vi "Change Type.vi"(8 "error in (no error)":errorcluster, 10 "Type":i32(listbox), 11 "Numeric Data Type in":refnum<class "Numeric Data Type.lvclass">) -> (0 "error out":errorcluster, 3 "Numeric Data Type out":refnum<class "Numeric Data Type.lvclass">)   [LabVIEW 2018, in "Numeric Data Type.lvclass"]
uses:
  Numeric Data Type.lvclass
  Numeric Format Enum.ctl
  Numeric Data Type.lvclass/Numeric Data Type.ctl
  Numeric Info.ctl
  Precision Type.ctl
  Padding.ctl
  Time Info.ctl
  Time Format.ctl
  Clock Type.ctl
  Date Order.ctl
  Date Format.ctl
  Year Format.ctl
  Format Code Type List Enum.ctl
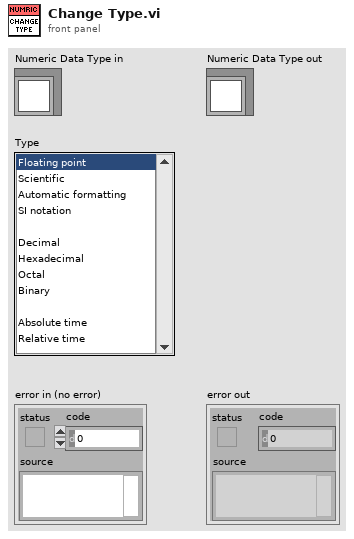
[diagram p1: front panel]
types:
  T1 = typedef "Numeric Data Type.lvclass/Numeric Format Enum.ctl" = enum16{"Floating Point Notation", "Scientific Notation", "Engineering Notation", "SI Notation", "<not used>", "Decimal", "Hexadecimal", "Octal", "Binary", "<not used 2>", "Absolute Time", "Relative Time"}
  T2 = typedef "Numeric Data Type.lvclass/Format Code Type List Enum.ctl" = enum16{"Numeric format codes", "Relative time format codes", "Absolute time format codes"}
  T3 = typedef "Numeric Data Type.lvclass/Numeric Info.ctl" = cluster{"Minimum Field Width":i32, "Digits of Precision":i32, "Numeric Format":T1, "Precision Type":T4, "Hide trailing zeros":bool, "exponent":bool, "just/pad":T5, "Modifiers":string}
  T4 = typedef "Numeric Data Type.lvclass/Precision Type.ctl" = enum16{"Digits of precision", "Significant digits"}
  T5 = typedef "Numeric Data Type.lvclass/Padding.ctl" = enum16{"Pad with spaces on left", "Pad with spaces on right", "Pad with zeros on left"}
  T6 = typedef "Numeric Data Type.lvclass/Time Info.ctl" = cluster{"Time Format":T7, "Numeric Format":T1, "Clock Type":T8, "Include Seconds?":bool, "Seconds Precision":i16, "Date Order":T9, "Date Format":T10, "Year Format":T11, "UTC":i16}
  T7 = typedef "Numeric Data Type.lvclass/Time Format.ctl" = enum16{"Custom time format", "System time format", "Time unused"}
  T8 = typedef "Numeric Data Type.lvclass/Clock Type.ctl" = enum32{"12-Hour (AM/PM)", "24-Hour"}
  T9 = typedef "Numeric Data Type.lvclass/Date Order.ctl" = enum32{"M/D/Y", "D/M/Y", "Y/M/D"}
  T10 = typedef "Numeric Data Type.lvclass/Date Format.ctl" = enum16{"Custom date format", "System date format", "Date unused"}
  T11 = typedef "Numeric Data Type.lvclass/Year Format.ctl" = enum32{"No Year", "2-digit Year", "4-digit Year"}
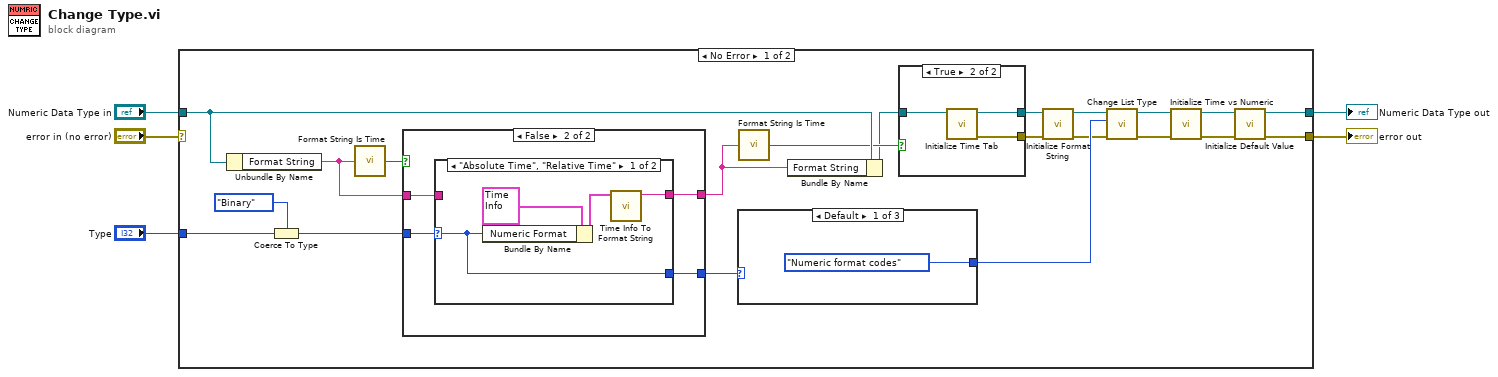
[diagram p0: block diagram]
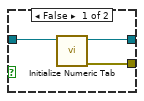
[diagram p2: hidden frame]
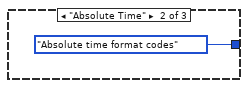
[diagram p3: hidden frame]
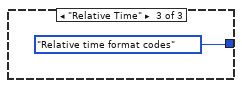
[diagram p4: hidden frame]
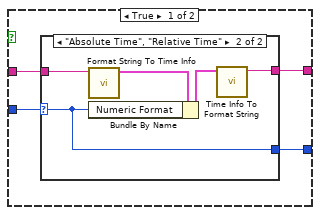
[diagram p5: hidden frame]
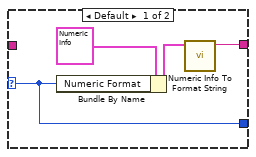
[diagram p6: hidden frame]
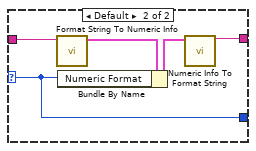
[diagram p7: hidden frame]
diagram:
  n1 = case shown="No Error" "error in (no error)" {
    selector: "error in (no error)" -> [_ w63]
    tunnel: [w9 w63] -> w4
    tunnel: [w11 w62] -> w2
    tunnel: "Numeric Data Type in" -> [w23 w62]
    tunnel: "Type" -> [w8 _]
    frame No Error {
      n2 = Unbundle By Name(w23) -> ("Format String"=w25:string)
      n3 = Coerce To Type(0:w8, 1:Numeric_Format_Enum."Binary" ("Numeric Format")) -> (2:w7:T1)
      n4 = call "Format String Is Time.vi"("Format String"=w25) -> ("Time?"=w26:bool)
      n5 = case shown="False" w26 {
        tunnel: w25 -> [w39 w52]
        tunnel: w7 -> [w37 w50]
        tunnel: [w38 w51] -> w19
        tunnel: [w36 w49] -> w24
        frame True {
          n6 = case shown="\"Absolute Time\", \"Relative Time\"" w37 {
            selector: w37 -> [w40 w44]
            tunnel: w39 -> [_ w48]
            tunnel: [w41 w45] -> w38
            tunnel: [w40 w44] -> w36
            frame Default {
              n7 = Bundle By Name(cluster=T3 {"Minimum Field Width"=0, "Digits of Precision"=0, "Numeric Format"=enum."Floating Point Notation", "Precision Type"=enum."Digits of precision", "Hide trailing zeros"=FALSE, "exponent"=FALSE, "just/pad"=enum."Pad with spaces on left", "Modifiers"=""} ("Numeric Format & Precision Info"), "Numeric Format"=w40) -> (w42:T3)
              n8 = call "Numeric Info To Format String.vi"("Numeric Format & Precision Info"=w42) -> ("Format String"=w41:string)  [unwired: 10 in]
            }
            frame "Absolute Time", "Relative Time" {
              n9 = call "Format String To Time Info.vi"("Format String"=w48) -> ("Time Info"=w47:T6)  [unwired: 10 in]
              n10 = Bundle By Name(cluster=w47, "Numeric Format"=w44) -> (w46:T6)
              n11 = call "Time Info To Format String.vi"("Time Format & Precision Info"=w46) -> ("Format String"=w45:string)  [unwired: 10 in]
            }
          }
        }
        frame False {
          n12 = case shown="\"Absolute Time\", \"Relative Time\"" w50 {
            selector: w50 -> [w53 w57]
            tunnel: w52 -> [_ w61]
            tunnel: [w54 w58] -> w51
            tunnel: [w53 w57] -> w49
            frame "Absolute Time", "Relative Time" {
              n13 = Bundle By Name(cluster=T6 {"Time Format"=enum."Custom time format", "Numeric Format"=enum."Floating Point Notation", "Clock Type"=enum."12-Hour (AM/PM)", "Include Seconds?"=FALSE, "Seconds Precision"=0, "Date Order"=enum."M/D/Y", "Date Format"=enum."Custom date format", "Year Format"=enum."No Year", "UTC"=0} ("Time Format & Precision Info"), "Numeric Format"=w53) -> (w56:T6)
              n14 = call "Time Info To Format String.vi"("Time Format & Precision Info"=w56) -> ("Format String"=w54:string)  [unwired: 10 in]
            }
            frame Default {
              n15 = call "Format String To Numeric Info.vi"("Format String"=w61) -> ("Numeric Format & Precision Info"=w60:T3)  [unwired: 10 in]
              n16 = Bundle By Name(cluster=w60, "Numeric Format"=w57) -> (w59:T3)
              n17 = call "Numeric Info To Format String.vi"("Numeric Format & Precision Info"=w59) -> ("Format String"=w58:string)  [unwired: 10 in]
            }
          }
        }
      }
      n18 = case shown="Default" w24 {
        tunnel: [Format_Code_Type_List_Enum."Numeric format codes" ("List type") Format_Code_Type_List_Enum."Absolute time format codes" ("List type") Format_Code_Type_List_Enum."Relative time format codes" ("List type")] -> w22
        frame Default {
        }
        frame "Absolute Time" {
        }
        frame "Relative Time" {
        }
      }
      n19 = call "Format String Is Time.vi"("Format String"=w19) -> ("Time?"=w18:bool)
      n20 = Bundle By Name(cluster=w23, "Format String"=w19) -> (w17:refnum<class "Numeric Data Type.lvclass">)
      n21 = case shown="True" w18 {
        tunnel: w17 -> [w29 w32]
        tunnel: [w28 w31] -> w16
        tunnel: [w27 w30] -> w15
        frame False {
          n22 = call "Initialize Numeric Tab.vi"("Numeric Data Type in"=w29) -> ("error out"=w27:errorcluster, "Numeric Data Type (dub)"=w28:refnum<class "Numeric Data Type.lvclass">)  [unwired: 9 in]
        }
        frame True {
          n23 = call "Initialize Time Tab.vi"("Numeric Data Type in"=w32) -> ("error out"=w30:errorcluster, "Numeric Data Type (dub)"=w31:refnum<class "Numeric Data Type.lvclass">)  [unwired: 9 in]
        }
      }
      n24 = call "Initialize Format String.vi"("error in (no error)"=w15, "Numeric Data Type in"=w16) -> ("error out"=w20:errorcluster, "Numeric Data Type (dup)"=w21:refnum<class "Numeric Data Type.lvclass">)  [unwired: 8 in]
      n25 = call "Change List Type.vi"("error in (no error)"=w20, "List type"=w22, "Numeric Data Type in"=w21) -> ("error out"=w13:errorcluster, "Numeric Data Type out"=w14:refnum<class "Numeric Data Type.lvclass">)  [unwired: 7 in]
      n26 = call "Initialize Time vs Numeric.vi"("error in (no error)"=w13, "Numeric Data Type in"=w14) -> ("error out"=w10:errorcluster, "Numeric Data Type (dup)"=w12:refnum<class "Numeric Data Type.lvclass">)  [unwired: 8 in]
      n27 = call "Initialize Default Value.vi"("error in (no error)"=w10, "Numeric Data Type in"=w12) -> ("error out"=w9:errorcluster, "Numeric Data Type (dup)"=w11:refnum<class "Numeric Data Type.lvclass">)  [unwired: 8 in]
    }
    frame Error {
    }
  }
  "error out" <- w4
  "Numeric Data Type out" <- w2
